vi "Conveyor and Shooter SS Implem.vi"(11 "Shooter and Conveyor Commands In":T1) -> (3 "Conveyor and Shooter Actuator Values Out":T2)   [LabVIEW 2016]
uses:
  Conveyor and Shooter Actuator Out.ctl
  Conveyor and Shooter Commands.ctl
  <vilib>/Rock Robotics/WPI/DriverStation/WPI_DriverStationRobotMode2.ctl
  Conveyor and Shoot Logging Values.vi
  Global Variables/Refnum Names.vi
  Global Variables/Conveyor Calibrations.vi
  Robot Global Data.vi
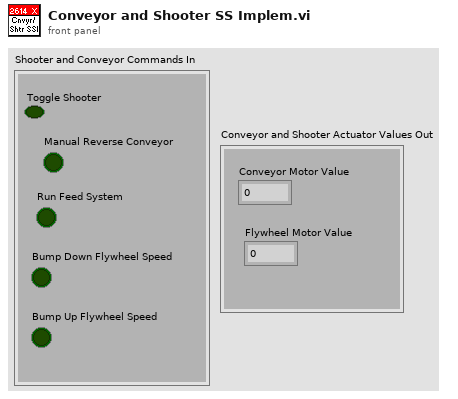
[diagram p1: front panel]
types:
  T1 = typedef "Conveyor and Shooter Commands.ctl" = cluster{"Toggle Shooter":bool, "Manual Reverse Conveyor":bool, "Run Feed System":bool, "Bump Down Flywheel Speed":bool, "Bump Up Flywheel Speed":bool}
  T2 = typedef "Conveyor and Shooter Actuator Out.ctl" = cluster{"Conveyor Motor Value":dbl, "Flywheel Motor Value":dbl}
  T3 = typedef "WPI_DriverStationRobotMode2.ctl" = enum16{"Autonomous Disabled", "Autonomous Enabled", "Teleop Disabled", "Teleop Enabled", "Disconnected", "Finish", "Test Disabled", "Test Enabled", "Emergency Stopped"}
  T4 = typedef "WPI_MotorControlDeviceRef.ctl" = cluster{"DeviceStatus":errorcluster, "Type":T5, "PWM":cluster{"PWM Channel":T6, "DeadBand":T7}, "CAN":cluster{"Device Number":u8, "SetOutput VI Ref":variant, "GetOutput VI Ref":variant, "Enable VI Ref":variant, "Disable VI Ref":variant, "Data":variant}, "Invert":bool}
  T5 = typedef "WPI_MotorControlType.ctl" = enum16{"PWM", "CAN"}
  T6 = typedef "FPGA_DIOPWMChannel.ctl" = enum8{"PWM 0", "PWM 1", "PWM 2", "PWM 3", "PWM 4", "PWM 5", "PWM 6", "PWM 7", "PWM 8", "PWM 9", "PWM MXP 0", "PWM MXP 1", "PWM MXP 2", "PWM MXP 3", "PWM MXP 4", "PWM MXP 5", "PWM MXP 6", "PWM MXP 7", "PWM MXP 8", "PWM MXP 9", "Invalid"}
  T7 = typedef "WPI_PWMDeadband.ctl" = cluster{"Name":string, "maxPositivePwm":i32, "minPositivePwm":i32, "centerPwm":i32, "maxNegativePwm":i32, "minNegativePwm":i32, "angularRange":u16}
  T8 = typedef "WPI_CANTalonSRX_GlobalStatus.ctl" = cluster{"Applied Throttle":dbl, "Module Enabled":bool, "CAN Error":errorcluster, "Closed Loop Error":dbl, "Forward Limit Switch Closed":bool, "Reverse Limit Switch Closed":bool, "Sensor Position":dbl, "Sensor Velocity":dbl, "Current":dbl, "Sticky Fault - Over Temp":bool, "Sticky Fault - Under Voltage":bool, "Sticky Fault - Forward Limit":bool, "Sticky Fault - Reverse Limit":bool, "Sticky Fault - Forward Soft Limit":bool, "Sticky Fault - Reverse Soft Limit":bool, "Brake is Enabled":bool, "Encoder Position":dbl, "Encoder Velocity":dbl, "Encoder Index Count":dbl, "Encoder A Pin State":bool, "Encoder B Pin State":bool, "Encoder Index Pin State":bool, "Analog In":dbl, "Analog In Velocity":dbl, "Temperature (C)":dbl, "Battery Voltage":dbl, "Control 5 Is Supported":bool, "Current Profile Slot Select":dbl, "Pos Div 8":bool, "Vel Div 4":bool, "Pulse Width Position":i32, "Pulse Width Velocity":i32, "Pulse Width Rise To Rise (us)":i32, "Pulse Width Rise To Fall (us)":i32, "Mot Prof Active Is Under Run":bool, "Mot Prof Active Has Under Run":bool, "Mot Prof Active Is Last":bool, "Mot Prof Active Velocity Only":bool, "Mot Prof Active Is Valid":bool, "Mot Prof Buffer Is Full":bool, "Mot Prof Active Profile Slot Select":i32, "Mot Prof NextID":i32, "Mot Prof Count":i32, "Mot Prof Active Velocity":dbl, "Mot Prof Active Position":dbl, "Mot Prof Output Enable":i32, "UsageFrame":u32, "Motion Magic Active Trajectory":cluster{"Velocity":dbl, "Position":dbl}}
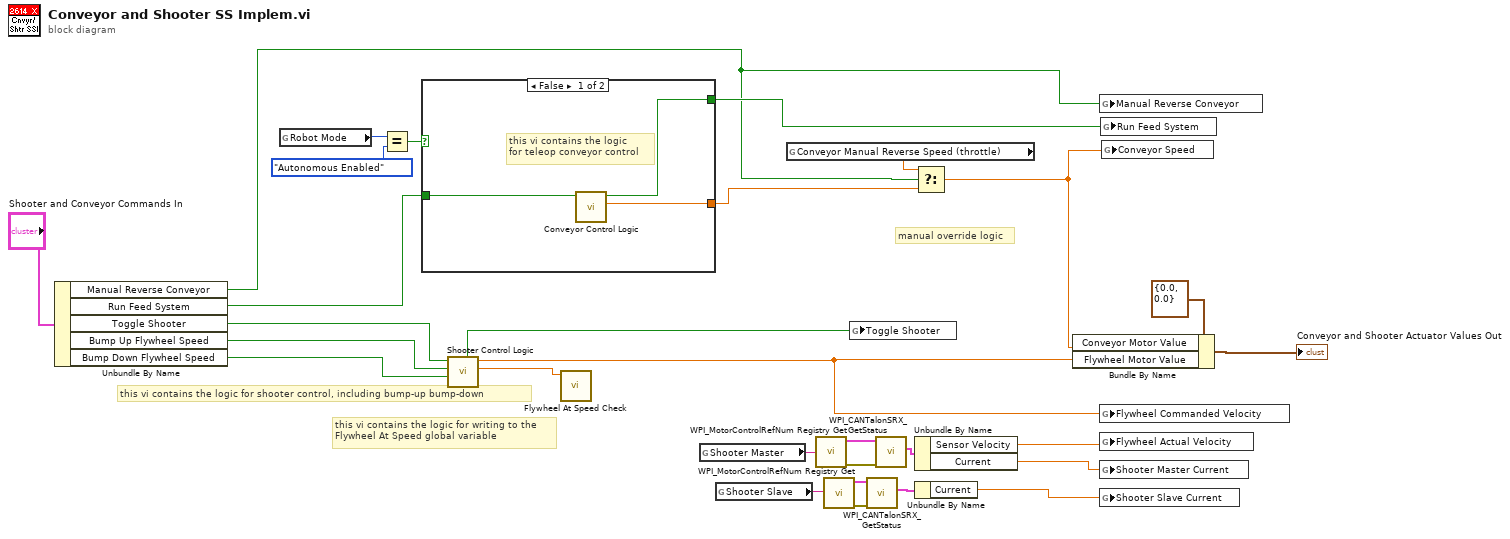
[diagram p0: block diagram]
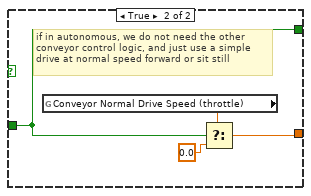
[diagram p2: hidden frame]
diagram:
  # "this vi contains the logic for writing to the\nFlywheel At Speed global variable"
  # "this vi contains the logic for shooter control, including bump-up bump-down"
  # "manual override logic"
  n1 = Unbundle By Name("Shooter and Conveyor Commands In") -> ("Manual Reverse Conveyor"=w6:bool, "Run Feed System"=w16:bool, "Toggle Shooter"=w12:bool, "Bump Up Flywheel Speed"=w11:bool, "Bump Down Flywheel Speed"=w10:bool)
  n2 = global read "Robot Global Data.vi" "Robot Mode"() -> (w15:T3)
  n3 = Equal?(x=w15, y=WPI_DriverStationRobotMode2."Autonomous Enabled" ("Robot Mode")) -> (x = y?=w13:bool)
  n4 = case shown="False" w13 {
    tunnel: [w32 w34] -> w17
    tunnel: [w31 w33] -> w7
    tunnel: w16 -> [w30 w33]
    frame False {
      # "this vi contains the logic\nfor teleop conveyor control"
      n5 = call "Conveyor Control Logic.vi"("Run Feed System In"=w30) -> ("Conveyor Motor Value Out"=w32:dbl, "Run Feed System Out"=w31:bool)  [unwired: 9 in]
    }
    frame True {
      # "if in autonomous, we do not need the other\nconveyor control logic, and just use a simple\ndrive at normal speed forward or sit still"
      n6 = global read "Conveyor Calibrations.vi" "Conveyor Normal Drive Speed (throttle)"() -> (w36:dbl)
      n7 = Select(t=w36, s=w33, f=0.0) -> (s? t:f=w34:dbl)
    }
  }
  n8 = call "Shooter Control Logic.vi"("Bump Down Flywheel Speed"=w10, "Bump Up Flywheel Speed"=w11, "Toggle Shooter In"=w12) -> ("Shooter Speed Calibration"=w9:dbl, "Commanded Shooter Speed"=w4:dbl, "Toggle Shooter Out"=w8:bool)  [unwired: 6 in]
  n9 = call "Flywheel At Speed Check.vi"("Shooter Speed Calibration"=w9) -> ()  [unwired: 11 in]
  n10 = global read "Refnum Names.vi" "Shooter Master"() -> (w24:string)
  n11 = global read "Refnum Names.vi" "Shooter Slave"() -> (w23:string)
  n12 = global read "Conveyor Calibrations.vi" "Conveyor Manual Reverse Speed (throttle)"() -> (w19:dbl)
  n13 = call <vilib>:"WPI_MotorControlRefNum Registry Get.vi"("refnum name"=w24) -> ("error out"=w27:errorcluster, "MotorControlDevRef"=w26:T4)  [unwired: 9 in]
  n14 = call <vilib>:"WPI_MotorControlRefNum Registry Get.vi"("refnum name"=w23) -> ("error out"=w20:errorcluster, "MotorControlDevRef"=w21:T4)  [unwired: 9 in]
  n15 = global write "Conveyor and Shoot Logging Values.vi" "Toggle Shooter"(w8) -> ()
  n16 = call <vilib>:"WPI_CANTalonSRX_GetStatus.vi"("error in (no error)"=w20, "CAN Talon SRX Ref"=w21) -> ("Talon SRX Status"=w22:T8)  [unwired: 7 in, 2 out]
  n17 = call <vilib>:"WPI_CANTalonSRX_GetStatus.vi"("error in (no error)"=w27, "CAN Talon SRX Ref"=w26) -> ("Talon SRX Status"=w25:T8)  [unwired: 7 in, 2 out]
  n18 = Unbundle By Name(w25) -> ("Sensor Velocity"=w3:dbl, "Current"=w2:dbl)
  n19 = Unbundle By Name(w22) -> ("Current"=w1:dbl)
  n20 = Select(t=w19, s=w6, f=w17) -> (s? t:f=w5:dbl)
  n21 = Bundle By Name(cluster=T2 {"Conveyor Motor Value"=0.0, "Flywheel Motor Value"=0.0} ("Conveyor and Shooter Actuator Values Out 2"), "Conveyor Motor Value"=w5, "Flywheel Motor Value"=w4) -> (→"Conveyor and Shooter Actuator Values Out":T2)
  n22 = global write "Conveyor and Shoot Logging Values.vi" "Manual Reverse Conveyor"(w6) -> ()
  n23 = global write "Conveyor and Shoot Logging Values.vi" "Flywheel Commanded Velocity"(w4) -> ()
  n24 = global write "Conveyor and Shoot Logging Values.vi" "Flywheel Actual Velocity"(w3) -> ()
  n25 = global write "Conveyor and Shoot Logging Values.vi" "Shooter Master Current"(w2) -> ()
  n26 = global write "Conveyor and Shoot Logging Values.vi" "Shooter Slave Current"(w1) -> ()
  n27 = global write "Conveyor and Shoot Logging Values.vi" "Run Feed System"(w7) -> ()
  n28 = global write "Conveyor and Shoot Logging Values.vi" "Conveyor Speed"(w5) -> ()
